vi "XY.vi"(0 "Y":dbl[](array[numeric]), 1 "X":dbl[](array[numeric])) -> ()   [LabVIEW 2014]
panel:
  out "XY Graph":cluster{"X":dbl[], "Y":dbl[]}(graph)
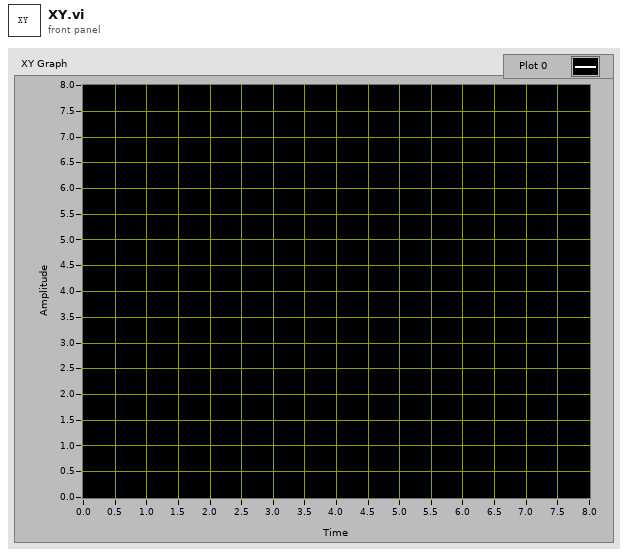
[diagram p1: front panel]
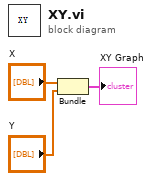
[diagram p0: block diagram]
diagram:
  n1 = Bundle("X"="X", "Y"="Y") -> (→"XY Graph":cluster{"X":dbl[], "Y":dbl[]})  [unwired: 1 in]
